vi "Sequence Commands.vi"(11 "queue in":refnum<queue>) -> ()   [LabVIEW 2025]
uses:
  23b8c87b-1961-4105-a430-c8e18ac4c775.vi
  751043b7-3e96-44c3-a3ec-d9298fca681b.vi
  <vilib>/Rock Robotics/WPI/DriverStation/WPI_DriverStationRobotMode2.ctl
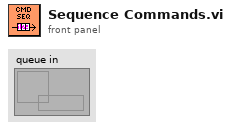
[diagram p1: front panel]
types:
  T1 = typedef "WPI_DriverStationRobotMode2.ctl" = enum16{"Autonomous Disabled", "Autonomous Enabled", "Teleop Disabled", "Teleop Enabled", "Disconnected", "Finish", "Test Disabled", "Test Enabled", "Emergency Stopped"}
  T2 = cluster{"Time (s)":dbl, "Command out":cluster{"Name":string, "vi reference":refnum<vi>, i32[], variant[]}}
  T3 = cluster{"Name":string, "vi reference":refnum<vi>, i32[], variant[]}
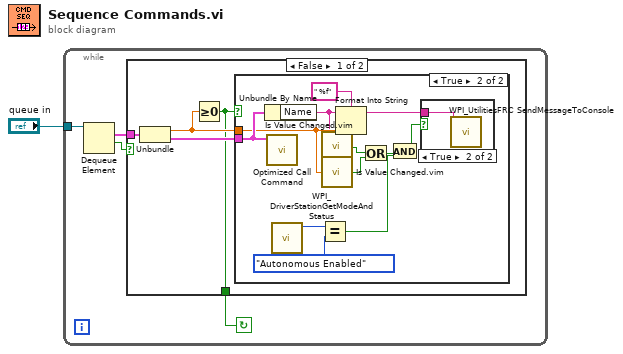
[diagram p0: block diagram]
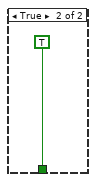
[diagram p4: hidden frame]
diagram:
  n1 = while {
    tunnel: "queue in" -> [w2]
    stop <- w3 continue-if-true
    n2 = Dequeue Element(queue=w2) -> (element=w5:T2, timed out?=w4:bool)  [unwired: 2 in, 2 out]
    n3 = case shown="False" w4 {
      tunnel: w5 -> [w9 _]
      tunnel: [w6 TRUE] -> w3
      frame False {
        n4 = Unbundle(w9) -> ("Time (s)"=w7:dbl, "Command out"=w8:T3)
        n5 = Greater Or Equal To 0?(x=w7) -> (x >= 0?=w6:bool)
        n6 = case shown="True" w6 {
          tunnel: w8 -> [_ w20]
          tunnel: w7 -> [_ w18]
          frame False {
          }
          frame True {
            n7 = Unbundle By Name(w20) -> ("Name"=w17:string)
            n8 = call "Optimized Call Command.vi"("Command"=w20) -> ()  [unwired: 10 in, 1 out]
            n9 = call <vilib>:"WPI_DriverStationGetModeAndStatus.vi"() -> ("Robot Mode"=w13:T1)  [unwired: 10 in, 1 out]
            n10 = Equal?(x=w13, y=WPI_DriverStationRobotMode2."Autonomous Enabled") -> (x = y?=w11:bool)
            n11 = call "Is Value Changed.vim"("value"=w17) -> ("changed or first call?"=w16:bool)
            n12 = call "Is Value Changed.vim"("value"=w18) -> ("changed or first call?"=w15:bool)
            n13 = Format Into String(format string=" %f", initial string=w17, w18) -> (resulting string=w19:string)  [unwired: 1 in, 1 out]
            n14 = Or(x=w16, y=w15) -> (x .or. y?=w14:bool)
            n15 = And(x=w14, y=w11) -> (x .and. y?=w10:bool)
            n16 = case shown="True" w10 {
              tunnel: w19 -> [_ w22]
              frame False {
              }
              frame True {
                n17 = call <vilib>:"WPI_UtilitiesFRC SendMessageToConsole.vi"("Message"=w22) -> ()  [unwired: 14 in, 1 out]
              }
            }
          }
        }
      }
      frame True {
      }
    }
  }
